vi "Write DAQmx task.vi"(8 "error in (no error)":errorcluster, 10 "DAQmx task":refnum<k21>, 11 "Motor-DAQmx in":refnum<class "Motor-DAQmx.lvclass">) -> (0 "error out":errorcluster, 3 "Motor-DAQmx out":refnum<class "Motor-DAQmx.lvclass">)   [LabVIEW 2013, in "PowderDeposition.lvlib" / "Motor-DAQmx.lvclass"]
uses:
  Motor-DAQmx.lvclass
  Motor-DAQmx.lvclass/Motor-DAQmx.ctl
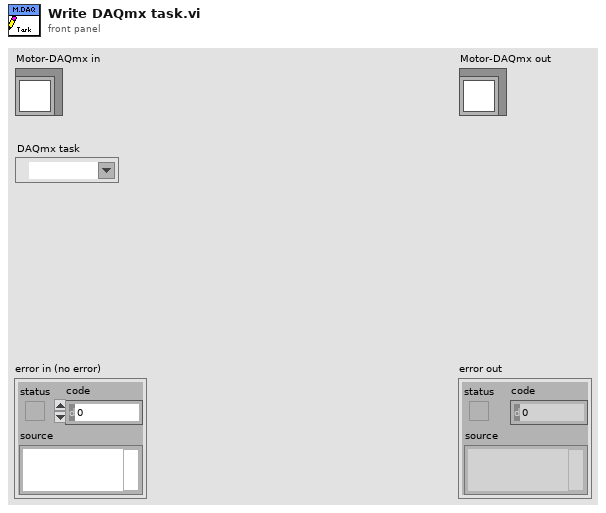
[diagram p1: front panel]
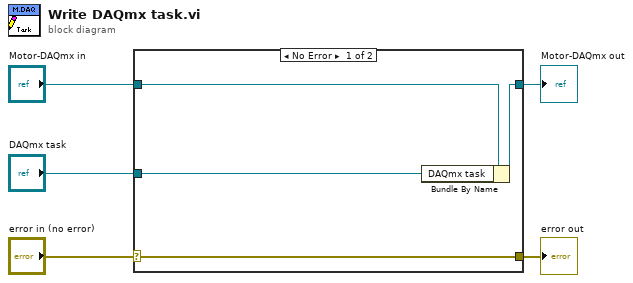
[diagram p0: block diagram]
diagram:
  n1 = case shown="No Error" "error in (no error)" {
    selector: "error in (no error)" -> [w9 w10]
    tunnel: [w9 w10] -> w4
    tunnel: [w7 w11] -> w2
    tunnel: "Motor-DAQmx in" -> [w8 w11]
    tunnel: "DAQmx task" -> [w6 _]
    frame No Error {
      n2 = Bundle By Name(cluster=w8, "DAQmx task"=w6) -> (w7:refnum<class "Motor-DAQmx.lvclass">)
    }
    frame Error {
    }
  }
  "error out" <- w4
  "Motor-DAQmx out" <- w2
